vi "ArduinoIDE.vi"() -> ()   [LabVIEW 2020]
panel:
  in  "OK Button":bool
  in  "File name":string
  in  "code":string
  in  "Link to Java Folder ... looks something like the link above":path
  out "Output":string
  out "Error":string
  # "/private/var/folders/26/wcn60znd5c3dj0jjxmkrhm7r0000gn/T/AppTranslocation/1E5965F9-C3B7-4B42-ADDE-BEF852C11FE0/d/Arduino.app/Contents/Java"
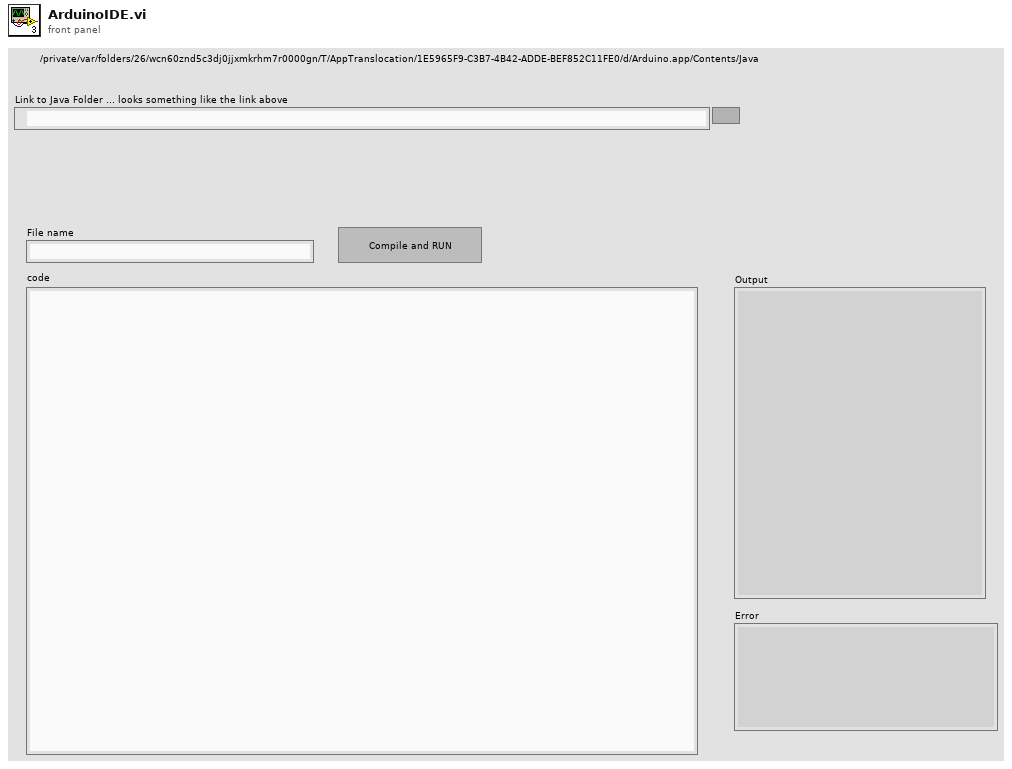
[diagram p1: front panel]
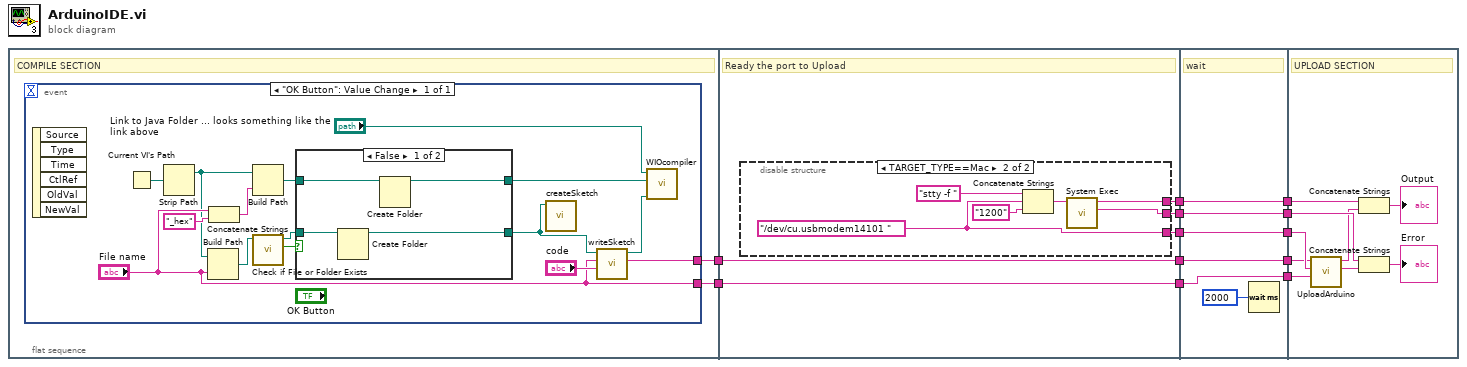
[diagram p0: block diagram]
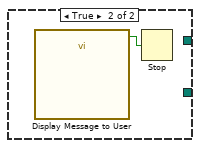
[diagram p2: hidden frame]
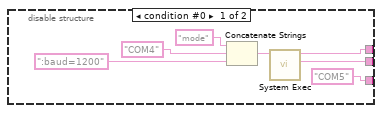
[diagram p3: hidden frame]
diagram:
  n1 = flat-sequence {
    tunnel: [w14] -> w6
    tunnel: [w13] -> w3
    tunnel: [w37] -> w12
    tunnel: [w38] -> w9
    tunnel: [w39] -> w8
    tunnel: w6 -> [w36]
    tunnel: [w36] -> w5
    tunnel: w3 -> [w35]
    tunnel: [w35] -> w2
    tunnel: w12 -> [w57]
    tunnel: [w57] -> w11
    tunnel: [w56] -> w10
    tunnel: w9 -> [w56]
    tunnel: w8 -> [w55]
    tunnel: [w55] -> w7
    tunnel: w5 -> [w54]
    tunnel: [w54] -> w4
    tunnel: w2 -> [w53]
    tunnel: [w53] -> w1
    tunnel: w11 -> [w61]
    tunnel: w10 -> [w67]
    tunnel: w7 -> [w64]
    tunnel: w4 -> [w60]
    tunnel: w1 -> [w59]
    frame #0 {
      # "COMPILE SECTION"
      n2 = event shown="[0] \"OK Button\": Value Change" {
        selector: _ -> [_]
        dyn-events: _ -> [_]
        timeout: _ -> [_]
        tunnel: [w23] -> w14
        tunnel: ["File name"] -> w13
        event "OK Button": Value Change {
          n3 = event-data() -> ()  [unwired: 1 in, 6 out]
          n4 = Current VI's Path() -> (path=w24:path)
          n5 = Strip Path(path=w24) -> (stripped path=w15:path)  [unwired: 1 out]
          n6 = Build Path(base path=w15, name or relative path="File name") -> (appended path=w27:path)
          n7 = Concatenate Strings("File name", "_hex" ("string")) -> (w19:string)
          n8 = Build Path(base path=w15, name or relative path=w19) -> (appended path=w18:path)
          n9 = call <vilib>:"Check if File or Folder Exists.vi"("path"=w27) -> ("file or folder exists?"=w28:bool, "dup path"=w25:path)  [unwired: 8 in, 1 out]
          n10 = case shown="False" w28 {
            tunnel: [w33 _] -> w26
            tunnel: w25 -> [w32 _]
            tunnel: w18 -> [w31 _]
            tunnel: [w30 _] -> w17
            frame False {
              n11 = Create Folder(path (use dialog)=w32) -> (created path=w33:path)  [unwired: 2 in, 2 out]
              n12 = Create Folder(path (use dialog)=w31) -> (created path=w30:path)  [unwired: 2 in, 2 out]
            }
            frame True {
              n13 = call "Display Message to User"() -> ("OK"=w34:bool)  [unwired: 10 in, 1 out]
              n14 = Stop(stop? (T)=w34) -> ()
            }
          }
          n15 = call "createSketch.vi"("path to ino folder"=w26) -> ()  [unwired: 10 in, 1 out]
          n16 = call "writeSketch.vi"("Code"="code", "File name"="File name", "path to ino folder"=w26) -> ("Sketch.ino"=w23:string, "path to ino file"=w21:path)  [unwired: 7 in]
          n17 = call "WIOcompiler.vi"("ino file"=w21, "hex folder"=w17, "Java"="Link to Java Folder ... looks something like the link above") -> ()  [unwired: 7 in, 2 out]
        }
      }
    }
    frame #1 {
      # "Ready the port to Upload"
      n18 = disable-structure shown="TARGET_TYPE==Mac" {
        disable-tunnel: [w42 w49] -> w39
        disable-tunnel: [w41 w48] -> w38
        disable-tunnel: ["COM5" ("string") w47] -> w37
        frame condition #0 {
          n19 = Concatenate Strings("mode" ("string"), "COM4" ("string"), ":baud=1200" ("string")) -> (w46:string)
          n20 = call <vilib>:"System Exec.vi"("command line"=w46) -> ("standard error"=w41:string, "standard output"=w42:string)  [unwired: 7 in, 2 out]
        }
        frame condition #1 (active) {
          w47 = "/dev/cu.usbmodem14101 " ("string")
          n21 = Concatenate Strings("stty -f " ("string"), w47, "1200" ("string")) -> (w52:string)
          n22 = call <vilib>:"System Exec.vi"("command line"=w52) -> ("standard error"=w48:string, "standard output"=w49:string)  [unwired: 7 in, 2 out]
        }
      }
    }
    frame #2 {
      # "wait"
      n23 = Wait (ms)(milliseconds to wait=u32 2000) -> ()  [unwired: 1 out]
    }
    frame #3 {
      # "UPLOAD SECTION"
      n24 = call "UploadArduino.vi"("sketch_hex"=w59, "serial port"=w61, "Sketch.ino"=w60) -> ("standard error"=w66:string, "standard output"=w63:string)  [unwired: 7 in]
      n25 = Concatenate Strings(w64, w63) -> (→"Output":string)
      n26 = Concatenate Strings(w67, w66) -> (→"Error":string)
    }
  }
